vi "Get LED States.vi"(8 "error in (no error)":errorcluster, 11 "LED Board Ref in":T2 format="%.0x") -> (0 "error out":errorcluster, 1 "Ordered LED Channels":T2[](array[typedef]) format="%.0x", 2 "LED States":T1[](array[typedef]), 3 "LED Board Ref out":T2 format="%.0x")   [LabVIEW 2014, in "SLSC configuration System Explorer.lvlib"]
doc: "Orders the fault channels and gets the current fault states of a single FIU board."
uses:
  SLSC configuration System Explorer.lvlib
  <vilib>/NI Veristand/Custom Device API/Custom Device Item Ref.ctl
  Shared/LED Backplane/LED State.ctl
  Shared/Constants.vi
  <vilib>/NI Veristand/Custom Device API/Get Item Property (U16).vi
  <vilib>/NI Veristand/Custom Device API/Custom Device API.lvlib
  Shared/SLSC configuration Shared.lvlib
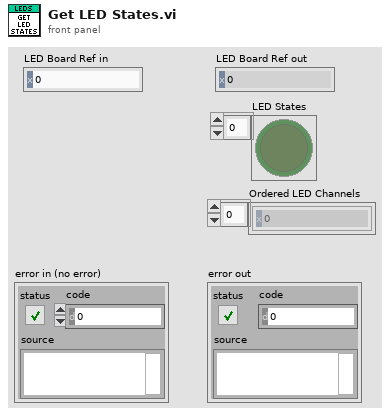
[diagram p1: front panel]
types:
  T1 = typedef "SLSC configuration Shared.lvlib/LED State.ctl" = bool
  T2 = typedef "Custom Device API.lvlib/Custom Device Item Ref.ctl" = u64
  T3 = typedef "Custom Device API.lvlib/Custom Device Channel.ctl" = cluster{"Type":T4, "Units":string, "Default Value":dbl, "Faultable":bool, "Scalable":bool}
  T4 = typedef "Custom Device API.lvlib/Custom Device Channel Type.ctl" = enum16{"Input", "Output"}
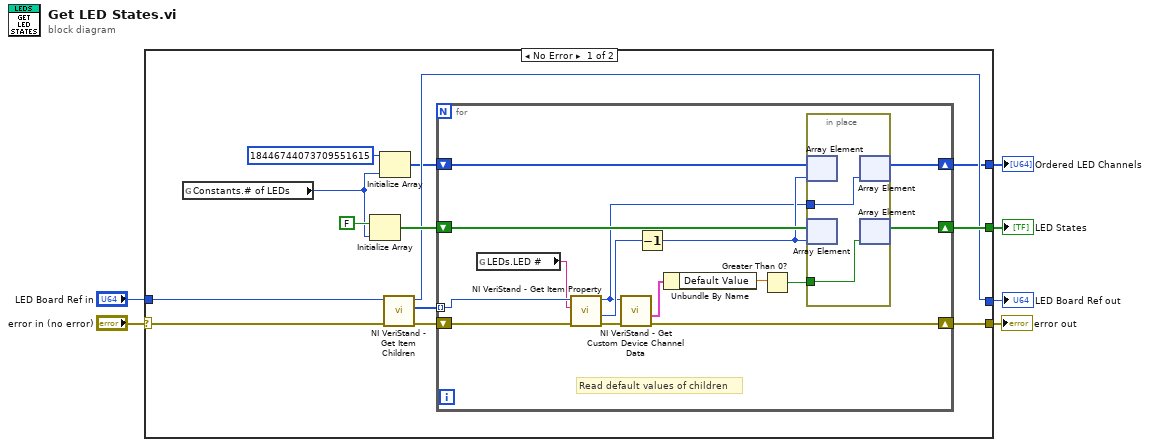
[diagram p0: block diagram]
diagram:
  n1 = case shown="No Error" "error in (no error)" {
    selector: "error in (no error)" -> [w12 w37]
    tunnel: "LED Board Ref in" -> [w17 w38]
    tunnel: [w16 w37] -> w5
    tunnel: [w13 _] -> w1
    tunnel: [w11 w38] -> w3
    tunnel: [w7 _] -> w2
    frame No Error {
      n2 = global read "Constants.vi" "Constants.# of LEDs"() -> (w9:u8)
      n3 = Initialize Array(T1 FALSE ("dimension size"), w9) -> (w19:T1[])
      n4 = Initialize Array(T2 18446744073709551615 ("Item Ref out"), w9) -> (w8:T2[])
      n5 = call <vilib>:"NI VeriStand - Get Item Children.vi"("error in (no error)"=w12, "Item Ref in"=w17) -> ("error out"=w15:errorcluster, "Child Refs"=w14:T2[], "Item Ref out"=w11:T2)  [unwired: 6 in, 1 out]
      n6 = for {
        tunnel: w14 -> [w34] mode=indexing
        shift-right: [w27] -> w16
        shift-left: w15 -> [w32]
        shift-right: [w26] -> w13
        shift-left: w19 -> [w28]
        shift-right: [w22] -> w7
        shift-left: w8 -> [w25]
        # "Read default values of children"
        n7 = global read "Constants.vi" "LEDs.LED #"() -> (w33:string)
        n8 = call-poly <vilib>:"NI VeriStand - Get Item Property.vi"("error in (no error)"=w32, "Property Name"=w33, "Item Ref in"=w34) -> ("error out"=w30:errorcluster, "Value"=w31:u16, "Item Ref out"=w23:T2)  [unwired: 5 in, 1 out]
        n9 = call <vilib>:"NI VeriStand - Get Custom Device Channel Data.vi"("error in (no error)"=w30, "Channel Ref in"=w23) -> ("error out"=w27:errorcluster, "Channel"=w29:T3)  [unwired: 4 in, 4 out]
        n10 = Decrement(x=w31) -> (x-1=w24:u16)
        n11 = Unbundle By Name(w29) -> ("Default Value"=w21:dbl)
        n12 = Greater Than 0?(x=w21) -> (x > 0?=w20:bool)
        n13 = in-place {
          in-place-border: w20 -> [w36]
          in-place-border: w23 -> [w35]
          n14 = in-place-array #1(w25, w24) -> ()  [unwired: 1 out]
          n15 = in-place-array #2(w28, w24) -> ()  [unwired: 1 out]
          n16 = in-place-array #1(w35) -> (w22:T2[])  [unwired: 1 out]
          n17 = in-place-array #2(w36) -> (w26:T1[])  [unwired: 1 out]
        }
      }
    }
    frame Error {
    }
  }
  "error out" <- w5
  "LED Board Ref out" <- w3
  "Ordered LED Channels" <- w2
  "LED States" <- w1
